vi "call message.vi"(8 "error in":errorcluster, 10 "Parameters":string[](array[string]), 11 "method name":string) -> (0 "error out":errorcluster, 2 "length":i32, 3 "response":string)   [LabVIEW 2009]
doc: "Creates a method call message body from an array of XML-RPC formatted data"
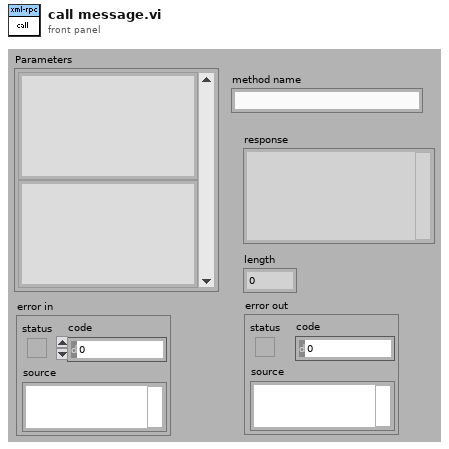
[diagram p1: front panel]
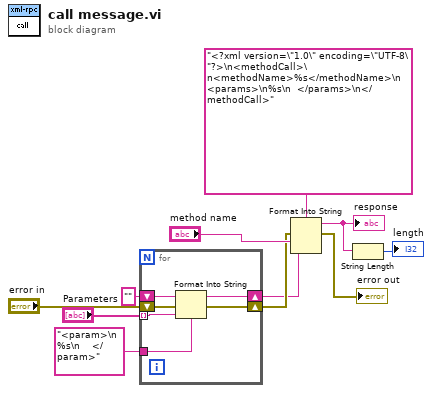
[diagram p0: block diagram]
diagram:
  n1 = for {
    tunnel: "Parameters" -> [w17] mode=indexing
    shift-right: [w15] -> w4
    shift-left: "error in" -> [w16]
    tunnel: "<param>\n      %s\n    </param>" ("format string") -> [w14]
    shift-right: [w13] -> w2
    shift-left: "" -> [w12]
    n2 = Format Into String(format string=w14, initial string=w12, error in=w16, w17) -> (resulting string=w13:string, error out=w15:errorcluster)
  }
  n3 = Format Into String(format string="<?xml version=\"1.0\" encoding=\"UTF-8\"?>\n<methodCall>\n<methodName>%s</methodName>\n  <params>\n%s\n  </params>\n</methodCall>", error in=w4, "method name", w2) -> (resulting string=w9:string, error out=→"error out":errorcluster)  [unwired: 1 in]
  "response" <- w9
  n4 = String Length(string=w9) -> (length=→"length":i32)
